vi "PurgeRequestWindow--Process.vi"(11 "TopLevel In":refnum<class "TopLevel.lvclass">) -> ()   [LabVIEW 2022 SP3, in "TopLevel.lvclass"]
uses:
  TopLevel.lvclass
  Icons/GreenControl_64.ctl
  Common/Controls/DLP_MaterialToHeadMapping--Cluster.ctl
  DLP2/DataTypes/DLP2_PrinterMaterialProperties.ctl
  Typedefs/InkIdleNodeConfigXML--Cluster.ctl
  Typedefs/InkProcessNodeConfigXML--Cluster.ctl
  Typedefs/PrimingMode APIData.ctl
  Typedefs/PurgeMode--Enum.ctl
  Typedefs/PrinterHeads--Enum.ctl
  DAQWFE/LV_Source/Subsystems/DAQ/DAQ.lvclass
panel:
  out "#":i32
  in  "Ignore":bool
  in  "PrintHead Wiped":bool
  out "Prime H 6":T1
  out "Prime H 5":T1
  out "Prime H 4":T1
  out "Prime H 3":T1
  out "Prime H 2":T1
  out "Prime H 1":T1
  out "TopLevel out":refnum<class "TopLevel.lvclass">
  in  "Purge":bool
  in  "OK":bool
  # "Idle Timer Expired. Prime may be required."
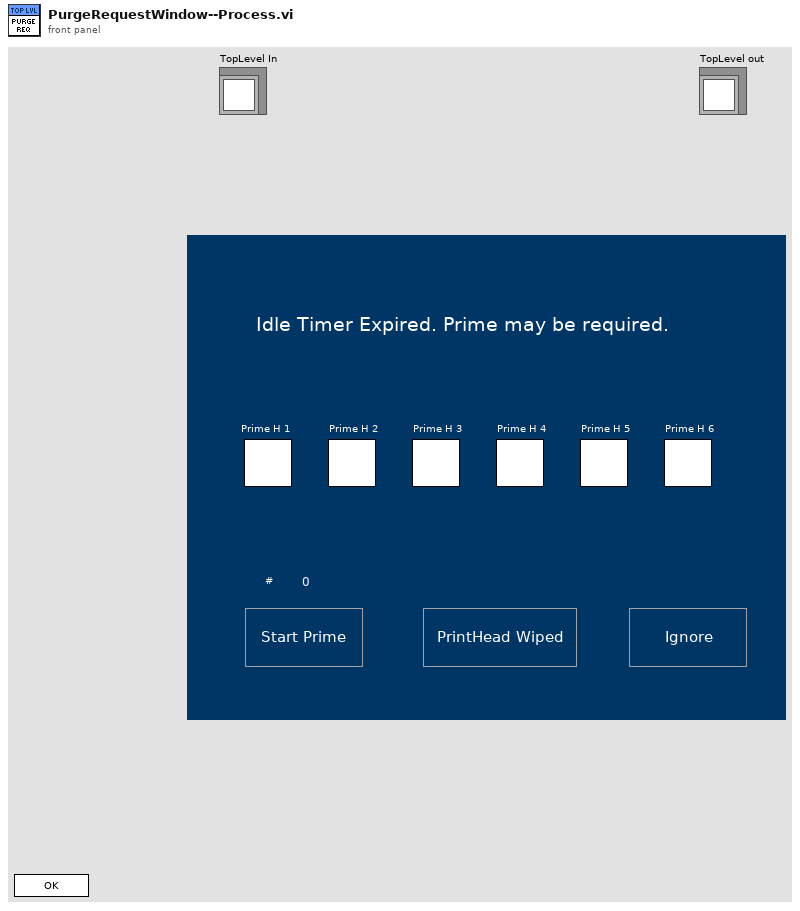
[diagram p1: front panel]
types:
  T1 = typedef "GreenControl_64.ctl" = bool
  T2 = enum32{"Invalid", "Standard", "Closed", "Hidden", "Minimized", "Maximized"}
  T3 = enum32{"invalid app kind", "Development System", "Run Time System", "Student Edition", "Embedded LabVIEW", "Evaluation", "Custom"}
  T4 = typedef "DLP_MaterialToHeadMapping--Cluster.ctl" = cluster{"Head":u8, "Ink":T5}
  T5 = typedef "DLP2_PrinterMaterialProperties.ctl" = cluster{"#attributes":cluster{"InkType":string, "PrePrintPurge":bool, "PurgeTime":dbl, "PurgeCount":i32, "Density":dbl, "NumberofDrops":i32, "PrintWeight":dbl, "PrintheadPrime":bool}, "Idle":T6, "Process":T7}
  T6 = typedef "InkIdleNodeConfigXML--Cluster.ctl" = cluster{"ShortIdle":cluster{"#attributes":cluster{"Heat":dbl, "Meniscus":dbl, "Recirculation":bool}}, "LongIdle":cluster{"#attributes":cluster{"Heat":dbl, "Meniscus":dbl, "Recirculation":bool}}}
  T7 = typedef "InkProcessNodeConfigXML--Cluster.ctl" = cluster{"C30_Process":cluster{"#attributes":cluster{"Heat":dbl, "Meniscus":dbl, "Recirculation":bool, "ColorPlane":string}}, "S30_Process":cluster{"#attributes":cluster{"Heat":dbl, "Meniscus":dbl, "Recirculation":bool, "ColorPlane":string}}}
  T8 = typedef "PurgeMode--Enum.ctl" = enum16{"Pre-Purge", "Purge", "Spit", "Shake"}
  T9 = typedef "DLPConfig_Initialization.ctl" = cluster{"PrinterInitialization":cluster{"Printer":cluster{"#attributes":cluster{"Name":string}}, "VacPumpSet":cluster{"#attributes":cluster{"VacPumpEnable":bool, "VacPumpSpeed":dbl}}, "HIBEnable":cluster{"#attributes":cluster{"HIB1Enable":bool, "HIB2Enable":bool, "HIB3Enable":bool, "HIB4Enable":bool, "HIB5Enable":bool, "HIB6Enable":bool}}, "PrinterCompensation":T10}, "HeadSet":cluster{"HeadProperties":T11[]}, "InkSet":cluster{"Ink":T5[]}, "Troubleshooting":cluster{"PMBLogging":cluster{"#attributes":cluster{"PMBMonitorDuringPrint":bool, "PMBMonitorDuringIdle":bool, "LogSwatheInputData":bool, "LogSwatheOutputData":bool, "LogPrintheadColourPlanes":bool, "LogPMBCommunication":bool, "LogSimulatedOutput":bool, "LogAllPMBCommunicationData":bool, "LogPMBSpace":bool, "ExtendedPMBSpaceLogging":bool, "LogPMBWriteSpeed":bool, "LogUsbRetries":bool}}, "HIBLogging":cluster{"#attributes":cluster{"HIBMonitoringDuringPrint":bool, "HIBMonitoringLog":bool}}}}
  T10 = typedef "DLP2_PrinterCompensationProperties.ctl" = cluster{"#attributes":cluster{"AppName":string, "PrintWeightMultiplier":dbl, "Rotation":bool, "Driver":string, "Server":string, "Database":string, "User":string, "Password":string}}
  T11 = typedef "DLP2_PrinterHeadProperties.ctl" = cluster{"#attributes":T12}
  T12 = typedef "DLPConfig)Init_HeadPropertyAttr--Cluster.ctl" = cluster{"HeadNumber":u8, "Material":string, "HeadLocalX":dbl, "HeadLocalY":dbl, "HeadRotationAngle":dbl, "VH2L_Hi":dbl, "VH2R_Hi":dbl, "VH1LA_Hi":dbl, "VH1LB_Hi":dbl, "VH1RA_Hi":dbl, "VH1RB_Hi":dbl, "VH2L_Lo":dbl, "VH2R_Lo":dbl, "VH1LA_Lo":dbl, "VH1LB_Lo":dbl, "VH1RA_Lo":dbl, "VH1RB_Lo":dbl}
  T13 = cluster{"Core":cluster{"Current VI Reference":refnum<vi>, "Close Panel on Exit?":bool}, "Your Boolean data":bool, "TopLevel In":refnum<class "TopLevel.lvclass">, "Methods:Accessors:PrinterInitializationXML":T9, "Methods:Accessors:DAQ":refnum<class "DAQ.lvclass">, "Array":u8[], "PrimeCnt":i32}
  T14 = cluster{"Current VI Reference":refnum<vi>, "Close Panel on Exit?":bool}
  T15 = typedef "TD Dynamic CVT DVR--ref.ctl" = refnum<data-value>
  T16 = typedef "TopLevel.lvclass/PrimingMode APIData.ctl" = cluster{"Interval (s)":dbl, "PurgeDuration (s)":dbl, "Repeats":u8, "PrimingMode":T8, "Head":T17, "Frequency (Hz)":i32, "PrintWeight":dbl}
  T17 = typedef "PrinterHeads--Enum.ctl" = enum16{"-1", "1", "2", "3", "4", "5", "6"}
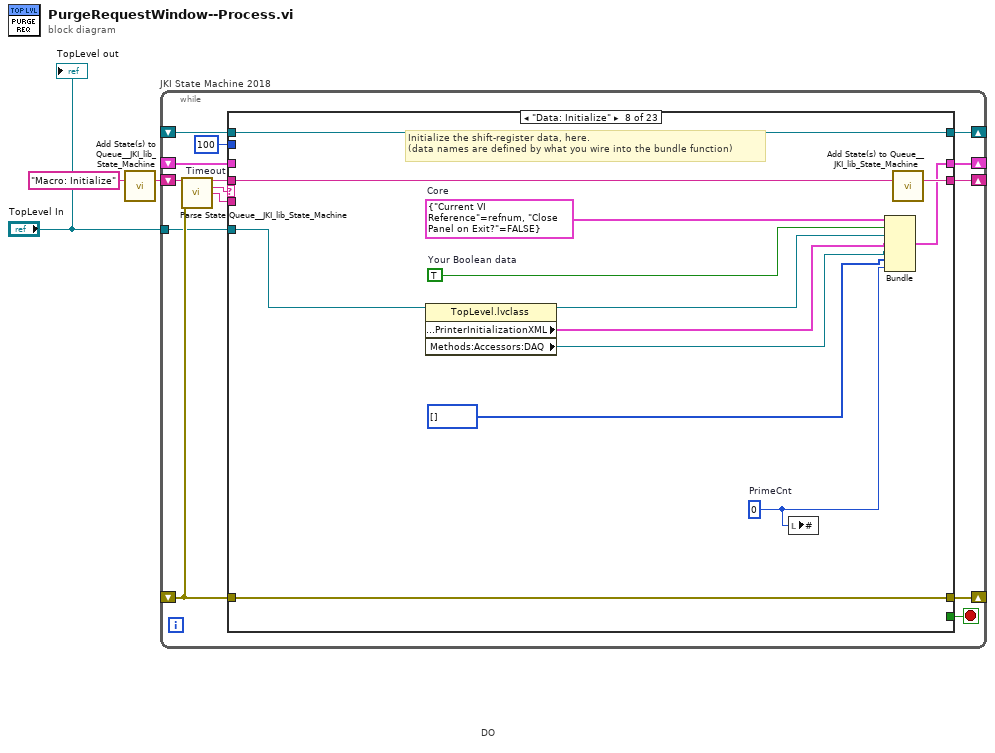
[diagram p0: block diagram]
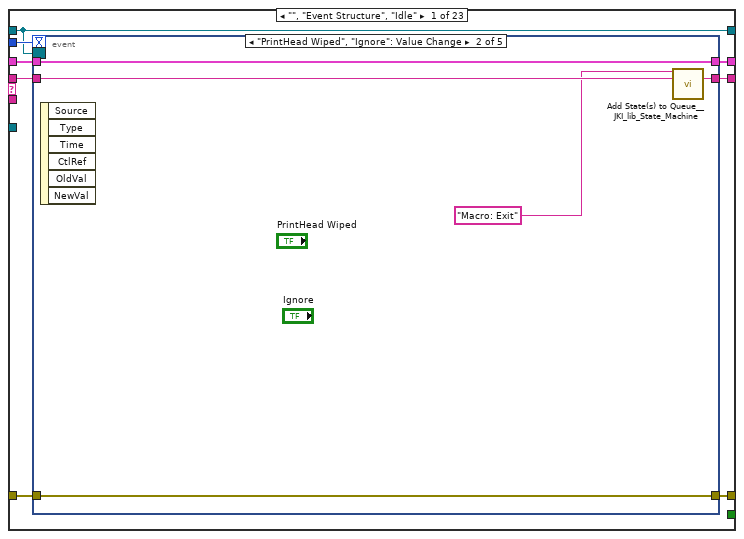
[diagram p2: hidden frame]
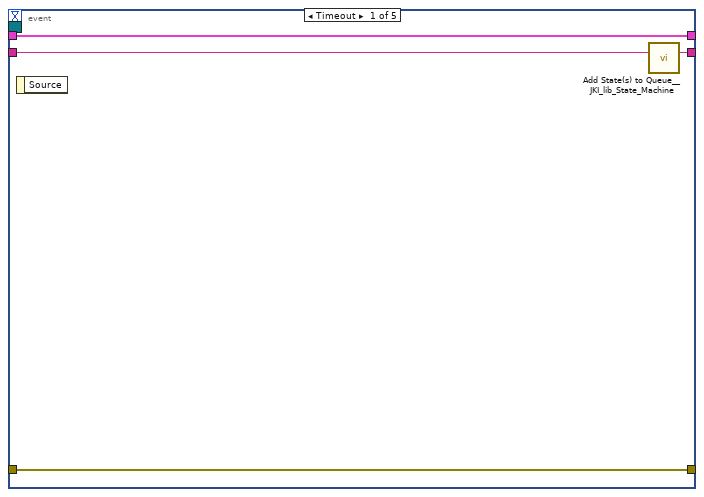
[diagram p3: hidden frame]
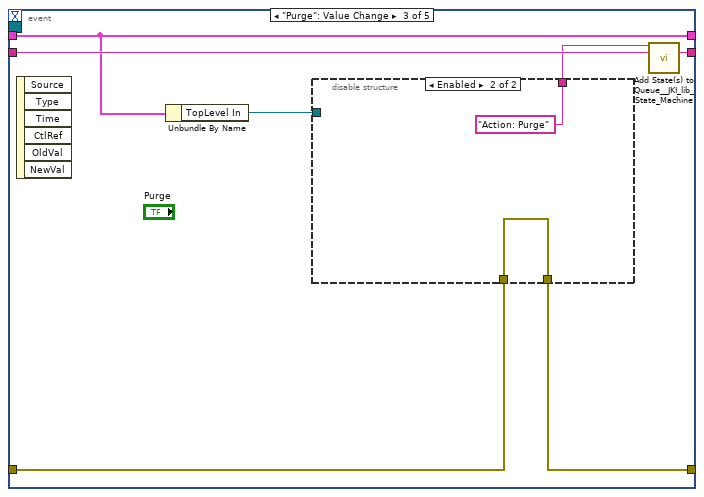
[diagram p4: hidden frame]
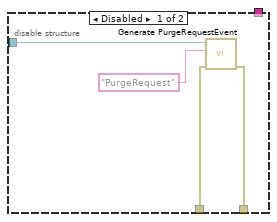
[diagram p5: hidden frame]
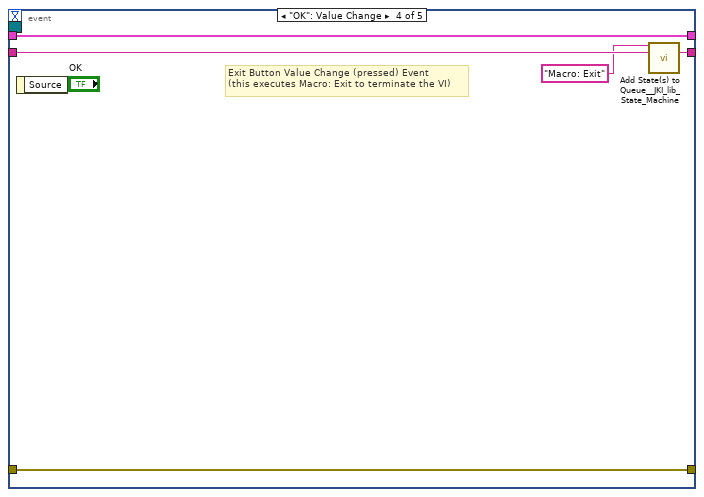
[diagram p6: hidden frame]
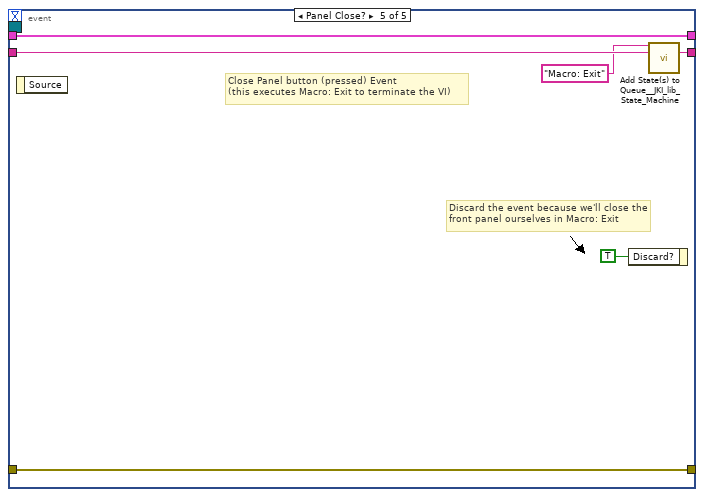
[diagram p7: hidden frame]
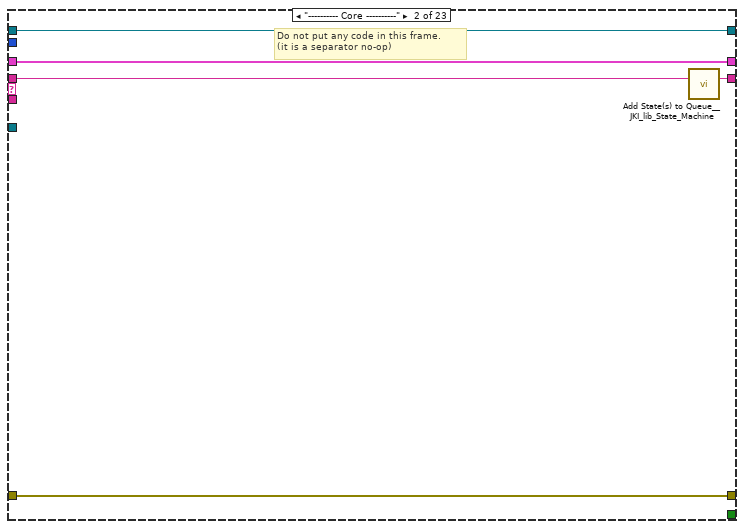
[diagram p8: hidden frame]
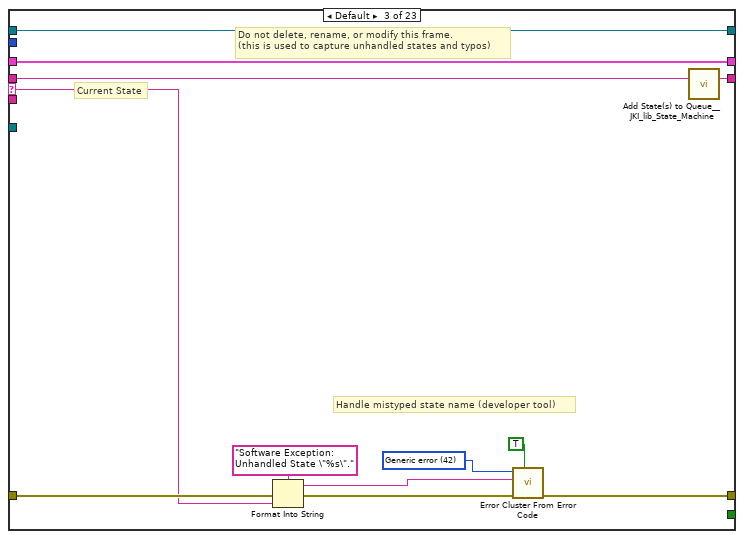
[diagram p9: hidden frame]
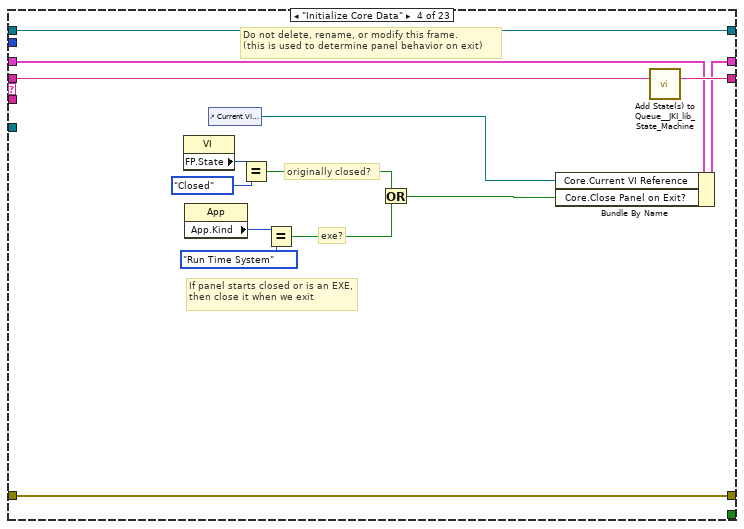
[diagram p10: hidden frame]
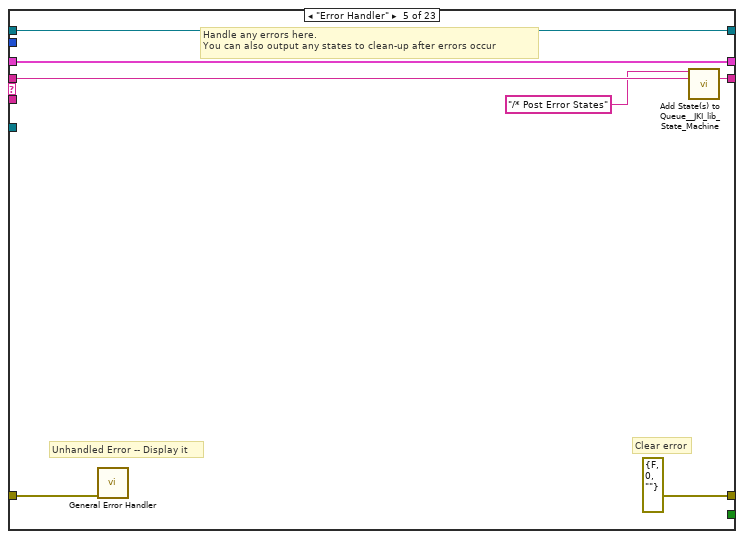
[diagram p11: hidden frame]
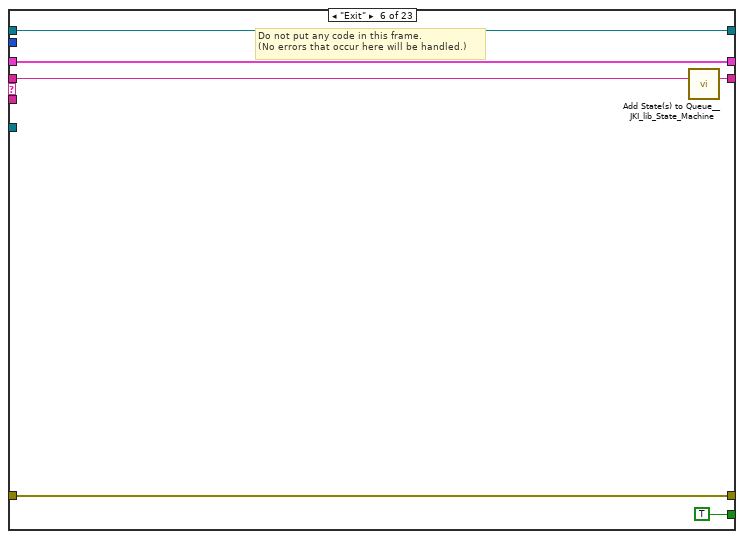
[diagram p12: hidden frame]
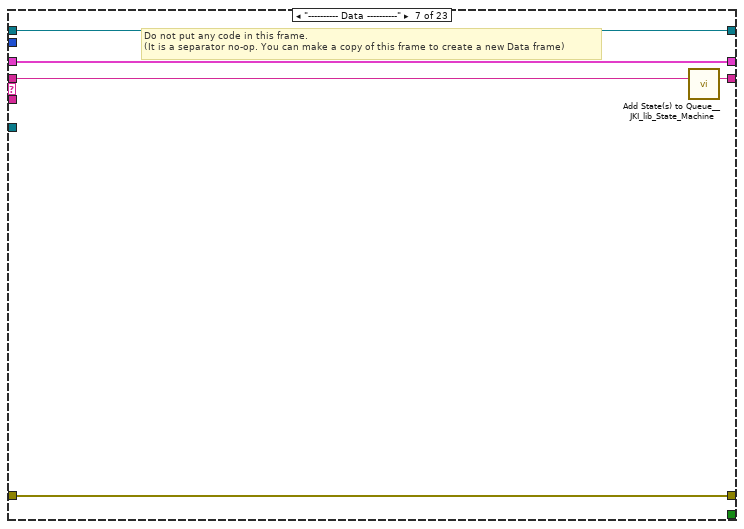
[diagram p13: hidden frame]
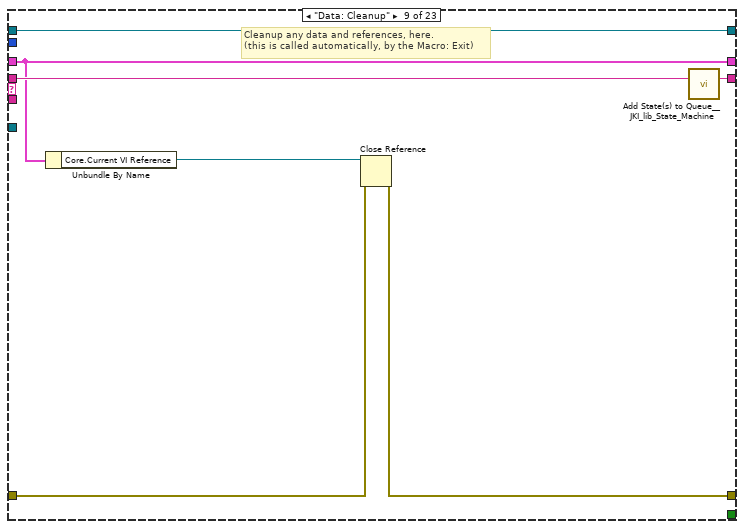
[diagram p14: hidden frame]
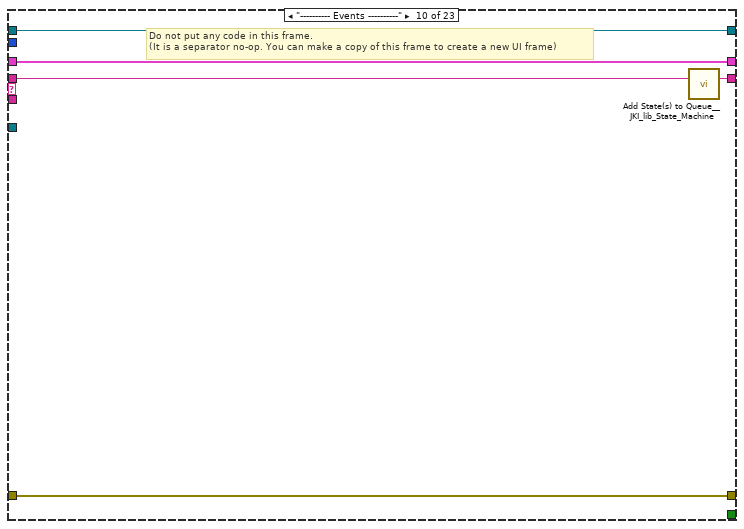
[diagram p15: hidden frame]
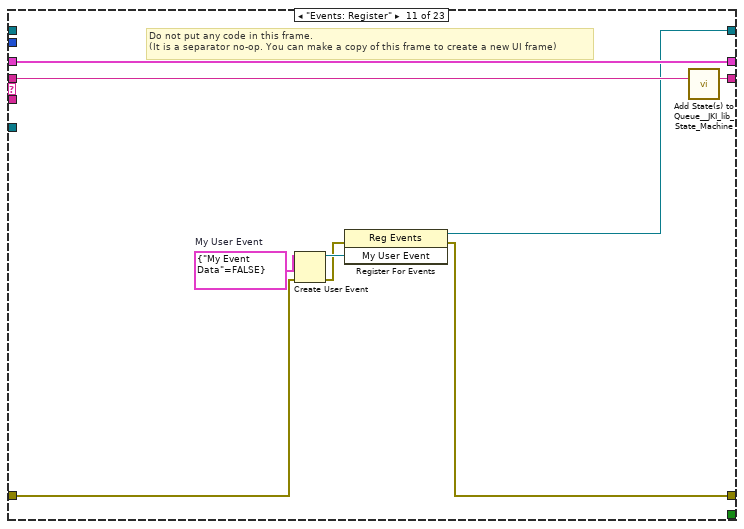
[diagram p16: hidden frame]
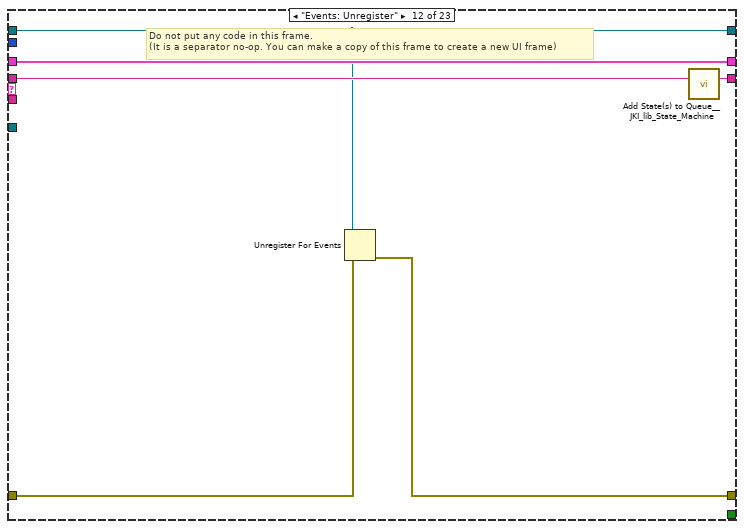
[diagram p17: hidden frame]
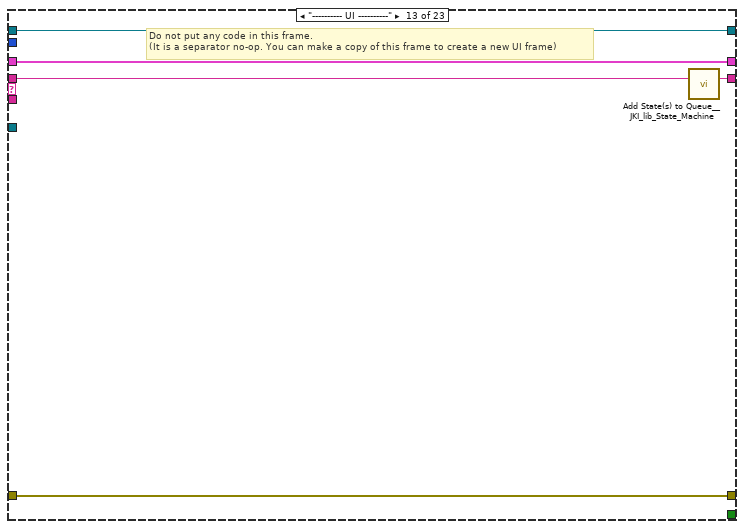
[diagram p18: hidden frame]
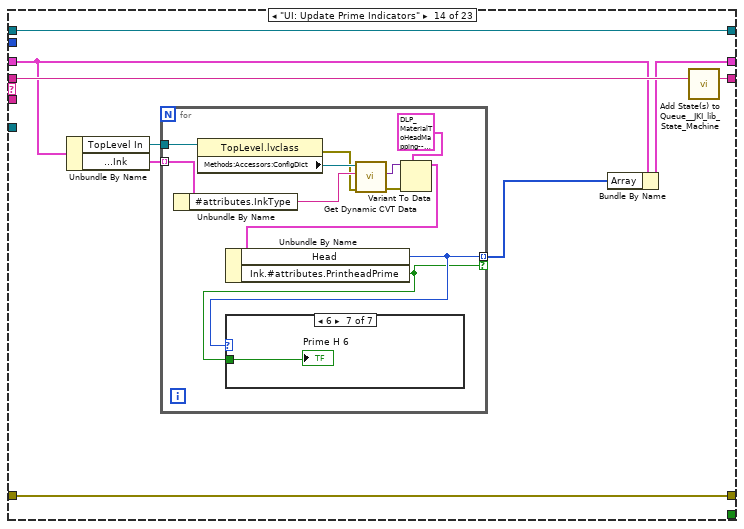
[diagram p19: hidden frame]
diagram:
  # "DO"
  n1 = call <vilib>:"Add State(s) to Queue__JKI_lib_State_Machine.vi"("State(s) in (\"\")"="Macro: Initialize") -> ("States Out"=w3:string)  [unwired: 14 in]
  n2 = while "JKI State Machine 2018" {
    shift-right: [w10] -> _
    shift-left: _ -> [w9]
    shift-right: [w13] -> _
    shift-left: _ -> [w7]
    shift-right: [w12] -> _
    shift-left: w3 -> [w14]
    shift-right: [w6] -> _
    shift-left: _ -> [w5]
    tunnel: "TopLevel In" -> [w4]
    stop <- w11 stop-if-true
    w8 = 100  # Timeout
    n3 = call <vilib>:"Parse State Queue__JKI_lib_State_Machine.vi"("State Queue"=w14, "Error In (no error)"=w7) -> ("Remaining States"=w16:string, "Current State"=w17:string, "Arguments"=w15:string)  [unwired: 11 in]
    n4 = case shown="\"Data: Initialize\"" w17 {
      selector: w17 -> [_ _ w65 _ _ _ _ _ _ _ _ _ _ _ _ _ _ _ _ _ _ _ _]
      tunnel: w16 -> [w25 w63 w69 w89 w96 w102 w107 w120 w127 w132 w141 w147 w152 w161 w184 w191 w203 w273 w279 w296 w301 w312 w346]
      tunnel: w15 -> [_ _ _ _ _ _ _ _ _ _ _ _ _ _ _ w186 w197 _ _ _ _ _ _]
      tunnel: w9 -> [w23 w60 w67 w82 w93 w100 w104 _ w122 w129 w139 w145 w149 w157 w182 w189 w199 w270 w276 w294 w298 w309 w343]
      tunnel: [w22 w61 w71 w86 errorcluster {"status"=FALSE, "code"=0, "source"=""} ("error out") w99 w105 w117 w123 w130 w133 w142 w150 w159 w180 w187 w200 w271 w277 w280 w299 w307 w344] -> w13
      tunnel: w7 -> [w21 w61 w70 w86 w92 w99 w105 w117 w124 w130 w135 w143 w150 w159 w179 w188 w201 w271 w277 w284 w299 w306 w344]
      tunnel: [w24 w62 w68 w88 w95 w101 w106 w119 w126 w131 w140 w146 w151 w160 w183 w190 w202 w272 w278 w295 w300 w311 w345] -> w12
      tunnel: [_ _ _ _ _ TRUE _ _ _ _ _ _ _ _ _ _ _ _ _ _ _ _ _] -> w11
      tunnel: [w20 w60 w67 w87 w93 w100 w104 w118 w122 w129 w139 w145 w149 w154 w182 w189 w199 w270 w276 w294 w298 w303 w343] -> w10
      tunnel: w8 -> [w19 _ _ _ _ _ _ _ _ _ _ _ _ _ _ _ _ _ _ _ _ _ _]
      tunnel: [w18 w59 w64 w76 w90 w97 w103 w114 w121 w128 w136 w144 w148 w158 w181 w185 w196 w269 w274 w287 w297 w310 w342] -> w6
      tunnel: w5 -> [w18 w59 w64 w76 w90 w97 w103 w114 w121 w128 _ w144 w148 w158 w181 w185 w196 w269 w274 w287 w297 w310 w342]
      tunnel: w4 -> [_ _ _ _ _ _ _ w113 _ _ _ _ _ _ _ _ _ _ _ _ _ _ _]
      frame "", "Event Structure", "Idle" {
        n5 = event shown="[1] \"PrintHead Wiped\", \"Ignore\": Value Change" {
          selector: w18 -> [_ _ _ _ _]
          dyn-events: _ -> [_ _ _ _ _]
          timeout: w19 -> [_ _ _ _ _]
          tunnel: w25 -> [w29 w34 w41 w52 w58]
          tunnel: [w28 w33 w40 w51 w57] -> w24
          tunnel: w23 -> [w26 w31 w39 w49 w55]
          tunnel: [w27 w32 w37 w50 w56] -> w22
          tunnel: w21 -> [w27 w32 w36 w50 w56]
          tunnel: [w26 w31 w39 w49 w55] -> w20
          event Timeout {
            n6 = event-data() -> ()  [unwired: 1 in, 1 out]
            n7 = call <vilib>:"Add State(s) to Queue__JKI_lib_State_Machine.vi"("State(s) in (\"\")"=w29) -> ("States Out"=w28:string)  [unwired: 14 in]
          }
          event "PrintHead Wiped", "Ignore": Value Change {
            n8 = event-data() -> ()  [unwired: 1 in, 6 out]
            n9 = call <vilib>:"Add State(s) to Queue__JKI_lib_State_Machine.vi"("State(s) in Front (\"\")"="Macro: Exit" ("State(s) in Front (\"\")"), "State(s) in (\"\")"=w34) -> ("States Out"=w33:string)  [unwired: 13 in]
          }
          event "Purge": Value Change {
            n10 = event-data() -> ()  [unwired: 1 in, 6 out]
            n11 = Unbundle By Name(w39) -> ("TopLevel In"=w38:refnum<class "TopLevel.lvclass">)
            n12 = disable-structure shown="Enabled" {
              disable-tunnel: w38 -> [w45 _]
              disable-tunnel: [w44 w47] -> w37
              disable-tunnel: w36 -> [w43 w47]
              disable-tunnel: [_ "Action: Purge" ("Command")] -> w35
              frame Disabled {
                n13 = call-dynamic "Generate PurgeRequestEvent.vi"("error in (no error)"=w43, "Command"="PurgeRequest", "TopLevel in"=w45) -> ("error out"=w44:errorcluster)  [unwired: 7 in, 1 out]
              }
              frame Enabled {
              }
            }
            n14 = call <vilib>:"Add State(s) to Queue__JKI_lib_State_Machine.vi"("State(s) in Front (\"\")"=w35, "State(s) in (\"\")"=w41) -> ("States Out"=w40:string)  [unwired: 13 in]
          }
          event "OK": Value Change {
            # "Exit Button Value Change (pressed) Event\n(this executes Macro: Exit to terminate the VI)"
            n15 = event-data() -> ()  [unwired: 1 in, 1 out]
            n16 = call <vilib>:"Add State(s) to Queue__JKI_lib_State_Machine.vi"("State(s) in Front (\"\")"="Macro: Exit", "State(s) in (\"\")"=w52) -> ("States Out"=w51:string)  [unwired: 13 in]
          }
          event Panel Close? {
            # "Discard the event because we'll close the front panel ourselves in Macro: Exit"
            # "Close Panel button (pressed) Event\n(this executes Macro: Exit to terminate the VI)"
            n17 = event-data() -> ()  [unwired: 1 in, 1 out]
            n18 = event-data("Discard?"=TRUE) -> ()  [unwired: 1 in, 1 out]
            n19 = call <vilib>:"Add State(s) to Queue__JKI_lib_State_Machine.vi"("State(s) in Front (\"\")"="Macro: Exit", "State(s) in (\"\")"=w58) -> ("States Out"=w57:string)  [unwired: 13 in]
          }
        }
      }
      frame "---------- Core ----------" {
        # "Do not put any code in this frame.\n(it is a separator no-op)"
        n20 = call <vilib>:"Add State(s) to Queue__JKI_lib_State_Machine.vi"("State(s) in (\"\")"=w63) -> ("States Out"=w62:string)  [unwired: 14 in]
      }
      frame Default {
        w74 = 42 items=["No error", "Argument error", "Memory is full", "Out of zone", "End of file", "File already open", "Generic file I/O error", "File not found", "File permission error", "Disk is full", "Duplicate path", "Too many files open", "System feature not enabled", "Resource file not found", "Cannot add resource", "Resource not found", "Image not found", "Image memory error", "Pen does not exist", "Config type invalid", "Config token not found", "Config parse error", "Config memory error", "Bad external code format", "Bad external code offset", "External code not present", "Null window", "Destroy window error", "Null menu", "Print aborted", "Bad print record", "Print driver error", "Windows error during printing", "Memory error during printing", "Print dialog error", "Generic print error", "Invalid device refnum", "Device not found", "Device parameter error", "Device unit error", "Cannot open device", "Device call aborted", "Generic error", "Cancelled by user", "Object ID too low", "Object ID too high", "Object not in heap", "Unknown heap", "Unknown object (invalid DefProc)", "Unknown object (DefProc not in table)", "Message out of range", "Invalid (null) method", "Unknown message", "Manager call not supported", "Bad address", "Network operation in progress", "Network operation timed out", "Connection is busy", "Network attribute not supported", "Network error", "Address in use", "System out of memory", "Connection aborted", "Connection refused", "Not connected", "Already connected", "Connection closed", "Initialization error (interapplication manager)", "Bad occurrence", "Wait on unbound occurrence handler", "Occurrence queue overflow", "Datalog type conflict", "Unused", "Unrecognized type (interapplication manager)", "Memory corrupt", "Failed to make temporary DLL", "Old CIN version", "Drag socket not found", "Failed to load drop-object", "Failed to register OLE object", "Failed to release OLE object", "Format specifier type mismatch", "Unknown format specifier", "Too few format specifiers", "Too many format specifiers", "Scan failed", "Newer CIN version", "Error converting to variant", "Runtime menu error", "Password tampered", "Variant attribute not found", "Incompatible variant data type", "Event data is not available", "Event Store is not present", "Occurrence is not found", "Event Queue is not created", "Event info is not available", "Refnum passed is NULL", "Error retrieving Class GUID", "Error retrieving CoClass GUID", "Error retrieving TypeLib GUID.", "Bad built application magic bytes.", "Specific driver is different from the specific driver associated with the Logical Name.", "There is no session opened to the class driver.", "Max Error", "MAX - Error with config objects", "MAX - Error loading configuration", "MAX - Group not supported"]
        # "Current State"
        # "Do not delete, rename, or modify this frame.\n(this is used to capture unhandled states and typos)"
        # "Handle mistyped state name (developer tool)"
        n21 = Format Into String(format string="Software Exception: Unhandled State \"%s\"." ("message"), error in=w70, w65) -> (resulting string=w73:string, error out=w72:errorcluster)  [unwired: 1 in]
        n22 = call <vilib>:"Error Cluster From Error Code.vi"("show call chain? (False)"=TRUE, "error in (no error)"=w72, "error message (\"\")"=w73, "error code (0)"=w74) -> ("error out"=w71:errorcluster)  [unwired: 5 in]
        n23 = call <vilib>:"Add State(s) to Queue__JKI_lib_State_Machine.vi"("State(s) in (\"\")"=w69) -> ("States Out"=w68:string)  [unwired: 14 in]
      }
      frame "Initialize Core Data" {
        # "Do not delete, rename, or modify this frame.\n(this is used to determine panel behavior on exit)"
        # "originally closed?"
        # "exe?"
        # "If panel starts closed or is an EXE, then close it when we exit"
        n24 = property class="VI"() -> ("FP.State"=w79:T2)  [unwired: 2 in, 2 out]
        n25 = property class="App"() -> ("App.Kind"=w85:T3)  [unwired: 2 in, 2 out]
        n26 = control-ref of="Current VI Reference"() -> (w80:refnum<vi>)
        n27 = Equal?(x=w79, y=T2."Closed" ("Front Panel Window:State")) -> (x = y?=w77:bool)
        n28 = Equal?(x=w85, y=T3."Run Time System" ("Application:Kind")) -> (x = y?=w83:bool)
        n29 = Or(x=w77, y=w83) -> (x .or. y?=w81:bool)
        n30 = Bundle By Name(cluster=w82, "Core.Current VI Reference"=w80, "Core.Close Panel on Exit?"=w81) -> (w87:T13)
        n31 = call <vilib>:"Add State(s) to Queue__JKI_lib_State_Machine.vi"("State(s) in (\"\")"=w89) -> ("States Out"=w88:string)  [unwired: 14 in]
      }
      frame "Error Handler" {
        # "Unhandled Error -- Display it"
        # "Handle any errors here.\nYou can also output any states to clean-up after errors occur"
        # "Clear error"
        n32 = call <vilib>:"General Error Handler.vi"("error in (no error)"=w92) -> ()  [unwired: 10 in, 5 out]
        n33 = call <vilib>:"Add State(s) to Queue__JKI_lib_State_Machine.vi"("State(s) in Front (\"\")"="/* Post Error States", "State(s) in (\"\")"=w96) -> ("States Out"=w95:string)  [unwired: 13 in]
      }
      frame "Exit" {
        # "Do not put any code in this frame.\n(No errors that occur here will be handled.)"
        n34 = call <vilib>:"Add State(s) to Queue__JKI_lib_State_Machine.vi"("State(s) in (\"\")"=w102) -> ("States Out"=w101:string)  [unwired: 14 in]
      }
      frame "---------- Data ----------" {
        # "Do not put any code in this frame.\n(It is a separator no-op. You can make a copy of this frame to create a new Data frame)"
        n35 = call <vilib>:"Add State(s) to Queue__JKI_lib_State_Machine.vi"("State(s) in (\"\")"=w107) -> ("States Out"=w106:string)  [unwired: 14 in]
      }
      frame "Data: Initialize" {
        w108 = 0  # PrimeCnt
        w115 = T14 {"Current VI Reference"=refnum, "Close Panel on Exit?"=FALSE}  # Core
        w116 = TRUE  # Your Boolean data
        # "Initialize the shift-register data, here.\n(data names are defined by what you wire into the bundle function)"
        n36 = property class="TopLevel.lvclass"(reference=w113) -> (reference out=w112:refnum<class "TopLevel.lvclass">, "Methods:Accessors:PrinterInitializationXML"=w111:T9, "Methods:Accessors:DAQ"=w110:refnum<class "DAQ.lvclass">)  [unwired: 1 in, 1 out]
        n37 = local write "#"(w108) -> ()
        n38 = Bundle("Core"=w115, "Your Boolean data"=w116, "TopLevel In"=w112, "Methods:Accessors:PrinterInitializationXML"=w111, "Methods:Accessors:DAQ"=w110, "Array"=u8[] [], "PrimeCnt"=w108) -> (w118:T13)  [unwired: 1 in]
        n39 = call <vilib>:"Add State(s) to Queue__JKI_lib_State_Machine.vi"("State(s) in (\"\")"=w120) -> ("States Out"=w119:string)  [unwired: 14 in]
      }
      frame "Data: Cleanup" {
        # "Cleanup any data and references, here.\n(this is called automatically, by the Macro: Exit)"
        n40 = Unbundle By Name(w122) -> ("Core.Current VI Reference"=w125:refnum<vi>)
        n41 = Close Reference(reference=w125, error in (no error)=w124) -> (error out=w123:errorcluster)
        n42 = call <vilib>:"Add State(s) to Queue__JKI_lib_State_Machine.vi"("State(s) in (\"\")"=w127) -> ("States Out"=w126:string)  [unwired: 14 in]
      }
      frame "---------- Events ----------" {
        # "Do not put any code in this frame.\n(It is a separator no-op. You can make a copy of this frame to create a new UI frame)"
        n43 = call <vilib>:"Add State(s) to Queue__JKI_lib_State_Machine.vi"("State(s) in (\"\")"=w132) -> ("States Out"=w131:string)  [unwired: 14 in]
      }
      frame "Events: Register" {
        w137 = cluster{"My Event Data":bool} {"My Event Data"=FALSE}  # My User Event
        # "Do not put any code in this frame.\n(It is a separator no-op. You can make a copy of this frame to create a new UI frame)"
        n44 = Create User Event(user event datatype=w137, error in=w135) -> (user event=w138:refnum<user-event>, error out=w134:errorcluster)
        n45 = register-events(error in=w134, w138) -> (reference out=w136:refnum<event-registration>, error out=w133:errorcluster)  [unwired: 1 in]
        n46 = call <vilib>:"Add State(s) to Queue__JKI_lib_State_Machine.vi"("State(s) in (\"\")"=w141) -> ("States Out"=w140:string)  [unwired: 14 in]
      }
      frame "Events: Unregister" {
        # "Do not put any code in this frame.\n(It is a separator no-op. You can make a copy of this frame to create a new UI frame)"
        n47 = Unregister For Events(event registration refnum=w144, error in=w143) -> (error out=w142:errorcluster)
        n48 = call <vilib>:"Add State(s) to Queue__JKI_lib_State_Machine.vi"("State(s) in (\"\")"=w147) -> ("States Out"=w146:string)  [unwired: 14 in]
      }
      frame "---------- UI ----------" {
        # "Do not put any code in this frame.\n(It is a separator no-op. You can make a copy of this frame to create a new UI frame)"
        n49 = call <vilib>:"Add State(s) to Queue__JKI_lib_State_Machine.vi"("State(s) in (\"\")"=w152) -> ("States Out"=w151:string)  [unwired: 14 in]
      }
      frame "UI: Update Prime Indicators" {
        n50 = Unbundle By Name(w157) -> ("TopLevel In"=w156:refnum<class "TopLevel.lvclass">, "Methods:Accessors:PrinterInitializationXML.InkSet.Ink"=w155:T5[])
        n51 = for {
          tunnel: w156 -> [w172]
          tunnel: w155 -> [w170] mode=indexing
          tunnel: [w163] -> w153 mode=indexing if=w162
          n52 = Unbundle By Name(w170) -> ("#attributes.InkType"=w169:string)
          n53 = property class="TopLevel.lvclass"(reference=w172) -> (error out=w165:errorcluster, "Methods:Accessors:ConfigDict"=w171:T15)  [unwired: 1 in, 1 out]
          n54 = call <vilib>:"Get Dynamic CVT Data.vi"("error in (no error)"=w165, "DataName"=w169, "dCVT DVR"=w171) -> ("error out"=w166:errorcluster, "value"=w167:variant)  [unwired: 5 in, 2 out]
          n55 = Variant To Data(error in=w166, type=T4 {"Head"=0, "Ink"={"#attributes"={"InkType"="", "PrePrintPurge"=FALSE, "PurgeTime"=0.0, "PurgeCount"=0, "Density"=0.0, "NumberofDrops"=0, "PrintWeight"=0.0, "PrintheadPrime"=FALSE}, "Idle"={"ShortIdle"={"#attributes"={"Heat"=0.0, "Meniscus"=0.0, "Recirculation"=FALSE}}, "LongIdle"={"#attributes"={"Heat"=0.0, "Meniscus"=0.0, "Recirculation"=FALSE}}}, "Process"={"C30_Process"={"#attributes"={"Heat"=0.0, "Meniscus"=0.0, "Recirculation"=FALSE, "ColorPlane"=""}}, "S30_Process"={"#attributes"={"Heat"=0.0, "Meniscus"=0.0, "Recirculation"=FALSE, "ColorPlane"=""}}}}}, Variant=w167) -> (data=w164:T4)  [unwired: 1 out]
          n56 = Unbundle By Name(w164) -> ("Head"=w163:u8, "Ink.#attributes.PrintheadPrime"=w162:bool)
          n57 = case shown="6" w163 {
            tunnel: w162 -> [_ w173 w174 w175 w176 w177 w178]
            frame 0, Default {
            }
            frame 1 {
              "Prime H 1" <- w173
            }
            frame 2 {
              "Prime H 2" <- w174
            }
            frame 3 {
              "Prime H 3" <- w175
            }
            frame 4 {
              "Prime H 4" <- w176
            }
            frame 5 {
              "Prime H 5" <- w177
            }
            frame 6 {
              "Prime H 6" <- w178
            }
          }
        }
        n58 = Bundle By Name(cluster=w157, "Array"=w153) -> (w154:T13)
        n59 = call <vilib>:"Add State(s) to Queue__JKI_lib_State_Machine.vi"("State(s) in (\"\")"=w161) -> ("States Out"=w160:string)  [unwired: 14 in]
      }
      frame "UI: Initialize" {
        # "Initialize the User Interface, here.\n(this is called automatically, by the Macro: Init)"
        n60 = call <userlib>:"Fit VI window to Largest Dec__ogtk.vi"("error in (no error)"=w179) -> ("error out"=w180:errorcluster)  [unwired: 5 in, 1 out]
        n61 = call <vilib>:"Add State(s) to Queue__JKI_lib_State_Machine.vi"("State(s) in (\"\")"=w184) -> ("States Out"=w183:string)  [unwired: 14 in]
      }
      frame "UI: Cursor Set" {
        # "Argument"
        # "Set and Unset Cursor Busy.\n(Usage: \"UI: Cursor Set >> Busy|Idle\")"
        n62 = case shown="\"Idle\", Default" w186 {
          tunnel: w188 -> [w193 w195]
          tunnel: [w192 w194] -> w187
          frame "Idle", Default {
            n63 = call <vilib>:"Unset Busy.vi"("error in (no error)"=w193) -> ("error out"=w192:errorcluster)  [unwired: 10 in]
          }
          frame "Busy" {
            n64 = call <vilib>:"Set Busy.vi"("error in (no error)"=w195) -> ("error out"=w194:errorcluster)  [unwired: 9 in, 1 out]
          }
        }
        n65 = call <vilib>:"Add State(s) to Queue__JKI_lib_State_Machine.vi"("State(s) in (\"\")"=w191) -> ("States Out"=w190:string)  [unwired: 14 in]
      }
      frame "UI: Front Panel State" {
        # "Argument"
        # "Set Front Panel Open or Closed\n(Usage: \"UI: Front Panel State >> Open|Close\")"
        n66 = Unbundle By Name(w199) -> ("Core.Current VI Reference"=w198:refnum<vi>)
        n67 = case shown="\"Minimize\", \"Minimized\"" w197 {
          tunnel: w201 -> [w209 w224 w235 w248 w261]
          tunnel: [w211 w225 w237 w250 w263] -> w200
          tunnel: w198 -> [w210 w222 w236 w249 w262]
          frame "Open", "Standard", Default {
            w204 = T2."Standard" ("State")
            n68 = property class="VI"(reference=w210, error in=w209) -> (reference out=w207:refnum<vi>, error out=w208:errorcluster, "FP.State"=w206:T2)
            n69 = Not Equal?(x=w206, y=w204) -> (x != y?=w205:bool)
            n70 = case shown="True" w205 {
              tunnel: [w215 w217] -> w211
              tunnel: w208 -> [w214 w217]
              tunnel: w207 -> [w213 _]
              tunnel: w204 -> [w212 _]
              frame True {
                n71 = invoke class="VI" method="FP.Open"(reference=w213, error in=w214, "Activate"=TRUE, "State"=w212) -> (error out=w215:errorcluster)  [unwired: 1 in, 4 out]
              }
              frame False {
              }
            }
          }
          frame "Close", "Closed" {
            n72 = property class="VI"(reference=w222, error in=w224) -> (reference out=w221:refnum<vi>, error out=w223:errorcluster, "FP.State"=w219:T2)
            n73 = Not Equal?(x=w219, y=T2."Closed" ("Front Panel Window:State")) -> (x != y?=w218:bool)
            n74 = case shown="True" w218 {
              tunnel: [w226 w229] -> w225
              tunnel: w223 -> [w226 w228]
              tunnel: w221 -> [_ w227]
              frame False {
              }
              frame True {
                n75 = invoke class="VI" method="FP.Close"(reference=w227, error in=w228) -> (error out=w229:errorcluster)  [unwired: 1 in, 2 out]
              }
            }
          }
          frame "Hidden", "Hide" {
            w230 = T2."Hidden" ("State")
            n76 = property class="VI"(reference=w236, error in=w235) -> (reference out=w233:refnum<vi>, error out=w234:errorcluster, "FP.State"=w232:T2)
            n77 = Not Equal?(x=w232, y=w230) -> (x != y?=w231:bool)
            n78 = case shown="True" w231 {
              tunnel: [w241 w242] -> w237
              tunnel: w234 -> [w240 w242]
              tunnel: w233 -> [w239 _]
              tunnel: w230 -> [w238 _]
              frame True {
                n79 = invoke class="VI" method="FP.Open"(reference=w239, error in=w240, "State"=w238) -> (error out=w241:errorcluster)  [unwired: 2 in, 4 out]
              }
              frame False {
              }
            }
          }
          frame "Minimize", "Minimized" {
            w243 = T2."Minimized" ("State")
            n80 = property class="VI"(reference=w249, error in=w248) -> (reference out=w246:refnum<vi>, error out=w247:errorcluster, "FP.State"=w245:T2)
            n81 = Not Equal?(x=w245, y=w243) -> (x != y?=w244:bool)
            n82 = case shown="True" w244 {
              tunnel: [w254 w255] -> w250
              tunnel: w247 -> [w253 w255]
              tunnel: w246 -> [w252 _]
              tunnel: w243 -> [w251 _]
              frame True {
                n83 = invoke class="VI" method="FP.Open"(reference=w252, error in=w253, "State"=w251) -> (error out=w254:errorcluster)  [unwired: 2 in, 4 out]
              }
              frame False {
              }
            }
          }
          frame "Maximize", "Maximized" {
            w256 = T2."Maximized" ("State")
            n84 = property class="VI"(reference=w262, error in=w261) -> (reference out=w259:refnum<vi>, error out=w260:errorcluster, "FP.State"=w258:T2)
            n85 = Not Equal?(x=w258, y=w256) -> (x != y?=w257:bool)
            n86 = case shown="True" w257 {
              tunnel: [w267 w268] -> w263
              tunnel: w260 -> [w266 w268]
              tunnel: w259 -> [w265 _]
              tunnel: w256 -> [w264 _]
              frame True {
                n87 = invoke class="VI" method="FP.Open"(reference=w265, error in=w266, "State"=w264) -> (error out=w267:errorcluster)  [unwired: 2 in, 4 out]
              }
              frame False {
              }
            }
          }
        }
        n88 = call <vilib>:"Add State(s) to Queue__JKI_lib_State_Machine.vi"("State(s) in (\"\")"=w203) -> ("States Out"=w202:string)  [unwired: 14 in]
      }
      frame "---------- Macro ----------" {
        # "Do not put any code in this frame.\n(It is a separator no-op. You can make a copy of this frame to create a new Macro frame)"
        n89 = call <vilib>:"Add State(s) to Queue__JKI_lib_State_Machine.vi"("State(s) in (\"\")"=w273) -> ("States Out"=w272:string)  [unwired: 14 in]
      }
      frame "Macro: Initialize" {
        # "Initialization Macro\n(This is called once, when the VI starts)"
        n90 = call <vilib>:"Add State(s) to Queue__JKI_lib_State_Machine.vi"("State(s) in Front (\"\")"="Data: Initialize\nInitialize Core Data\nEvents: Register\nUI: Initialize\nUI: Front Panel State >> Open\nUI: Update Prime Indicators", "State(s) in (\"\")"=w279) -> ("States Out"=w278:string)  [unwired: 13 in]
      }
      frame "Macro: Exit" {
        # "Exit Macro\n(This is called once, when the VI exits)"
        n91 = Unbundle By Name(w294) -> ("Core.Close Panel on Exit?"=w293:bool, "Methods:Accessors:DAQ"=w286:refnum<class "DAQ.lvclass">, "TopLevel In"=w283:refnum<class "TopLevel.lvclass">)
        n92 = call "Generate Timer Event.vi"("error in (no error)"=w284, "CmdMsg"="Done", "DAQ"=w286) -> ("error out"=w281:errorcluster)  [unwired: 7 in, 1 out]
        n93 = call-dynamic "Generate PurgeRequestEvent.vi"("error in (no error)"=w281, "Command"="Done" ("CmdMsg"), "TopLevel in"=w283) -> ("error out"=w280:errorcluster)  [unwired: 7 in, 1 out]
        n94 = Select(t="UI: Front Panel State >> Close", s=w293, f="") -> (s? t:f=w290:string)
        n95 = call <vilib>:"Add State(s) to Queue__JKI_lib_State_Machine.vi"("State(s) in (\"\")"=w290, "State(s) at Back (\"\")"="Data: Cleanup\nEvents: Unregister\nExit") -> ("States Out"=w288:string)  [unwired: 13 in]
        n96 = call <vilib>:"Add State(s) to Queue__JKI_lib_State_Machine.vi"("State(s) in Front (\"\")"=w288, "State(s) in (\"\")"=w296) -> ("States Out"=w295:string)  [unwired: 13 in]
      }
      frame "---------- New Category ----------" {
        # "Template Separator\n(You can make a copy of, or modify, this frame)"
        n97 = call <vilib>:"Add State(s) to Queue__JKI_lib_State_Machine.vi"("State(s) in (\"\")"=w301) -> ("States Out"=w300:string)  [unwired: 14 in]
      }
      frame "Action: Purge" {
        (unwired) string[] ["StartPrime 1", "StartPrime 2", "StartPrime 3", "StartPrime 4", "StartPrime 5", "StartPrime 6"]
        # "Your code here.\n(You can make a copy of, or modify, this frame)"
        n98 = Unbundle By Name(w309) -> ("PrimeCnt"=w304:i32, "TopLevel In"=w308:refnum<class "TopLevel.lvclass">, "Array"=w305:u8[])
        n99 = for {
          tunnel: w308 -> [w319]
          tunnel: [w317] -> w307
          tunnel: w306 -> [w316]
          tunnel: w305 -> [w315] mode=indexing
          w323 = T16 {"Interval (s)"=0.1, "PurgeDuration (s)"=0.1, "Repeats"=0, "PrimingMode"=enum."Pre-Purge", "Head"=enum."-1", "Frequency (Hz)"=0, "PrintWeight"=0.1} ("Pre Purge API Data")
          n100 = call-dynamic "Read ConfigDict.vi"("error in (no error)"=w316, "TopLevel in"=w319) -> ("error out"=w322:errorcluster, "ConfigDIct"=w326:T15, "TopLevel out"=w320:refnum<class "TopLevel.lvclass">)  [unwired: 7 in]
          n101 = case shown="3" w315 {
            tunnel: ["Junk" "Prime 1" "Prime 2" "Prime 3" "Prime 4" "Prime 5" "Prime 6"] -> w314
            frame 0, Default {
            }
            frame 1 {
            }
            frame 2 {
            }
            frame 3 {
            }
            frame 4 {
            }
            frame 5 {
            }
            frame 6 {
            }
          }
          n102 = call <vilib>:"Get Dynamic CVT Data.vi"("error in (no error)"=w322, "default value (empty variant)"=w323, "DataName"=w314, "dCVT DVR"=w326) -> ("error out"=w325:errorcluster, "found"=w313:bool, "value"=w324:variant)  [unwired: 4 in, 1 out]
          n103 = Variant To Data(error in=w325, type=w323, Variant=w324) -> (data=w321:T16, error out=w318:errorcluster)
          n104 = case shown="True" w313 {
            tunnel: w321 -> [_ w334]
            tunnel: w320 -> [_ w331]
            tunnel: w318 -> [_ w328]
            tunnel: [_ w327] -> w317
            frame False {
            }
            frame True {
              n105 = Bundle By Name(cluster=w334, "PrimingMode"=PurgeMode--Enum."Purge", "Repeats"=u8 1) -> (w332:T16)
              n106 = call-dynamic "PrimeMode API.vi"("Wait (F)"=TRUE, "error in (no error)"=w328, "Pre Purge API Data"=w332, "TopLevel in"=w331) -> ("error out"=w327:errorcluster)  [unwired: 6 in, 1 out]
            }
          }
        }
        n107 = Increment(x=w304) -> (x+1=w302:i32)
        "#" <- w302
        n108 = Bundle By Name(cluster=w309, "PrimeCnt"=w302) -> (w303:T13)
        n109 = call <vilib>:"Add State(s) to Queue__JKI_lib_State_Machine.vi"("State(s) in (\"\")"=w312) -> ("States Out"=w311:string)  [unwired: 14 in]
      }
      frame "New Category: 2" {
        # "Your code here.\n(You can make a copy of, or modify, this frame)"
        n110 = call <vilib>:"Add State(s) to Queue__JKI_lib_State_Machine.vi"("State(s) in (\"\")"=w346) -> ("States Out"=w345:string)  [unwired: 14 in]
      }
    }
  }
  "TopLevel out" <- "TopLevel In"
